vi "Custom PID v1_1.vi"(1 "Anti-Windup":bool, 2 "Set Point":dbl format="%.3g", 3 "Present Value":dbl format="%.3f", 4 "Tuning Parameters":T1={"Controller Gain, Kc"=1.0, "Reset Time, Ti (s)"=0.01, "Derivative Time, Td (s)"=0.0} {"Derivative Time, Td (s)" format="%.3g"; "Reset Time, Ti (s)" format="%.3g"; "Controller Gain, Kc" format="%.3g"}) -> (0 "Controller Output":dbl format="%.3g")   [LabVIEW 2012]
uses:
  Global Variables PID.vi
panel:
  out "dt (min)":dbl format="%.3g"
  in  "dT (s)":dbl=-1.0 step=0.001 format="%.3f"
  # "This PID VI is meant to be used for instructional Purposes.  It is in ideal form and simplified down from the orginal PID VI from the default NI PID VI."
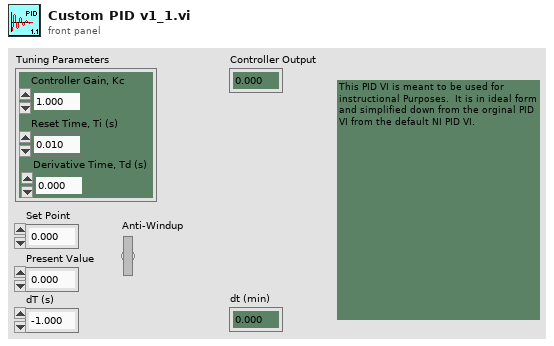
[diagram p1: front panel]
types:
  T1 = cluster{"Controller Gain, Kc":dbl, "Reset Time, Ti (s)":dbl, "Derivative Time, Td (s)":dbl}
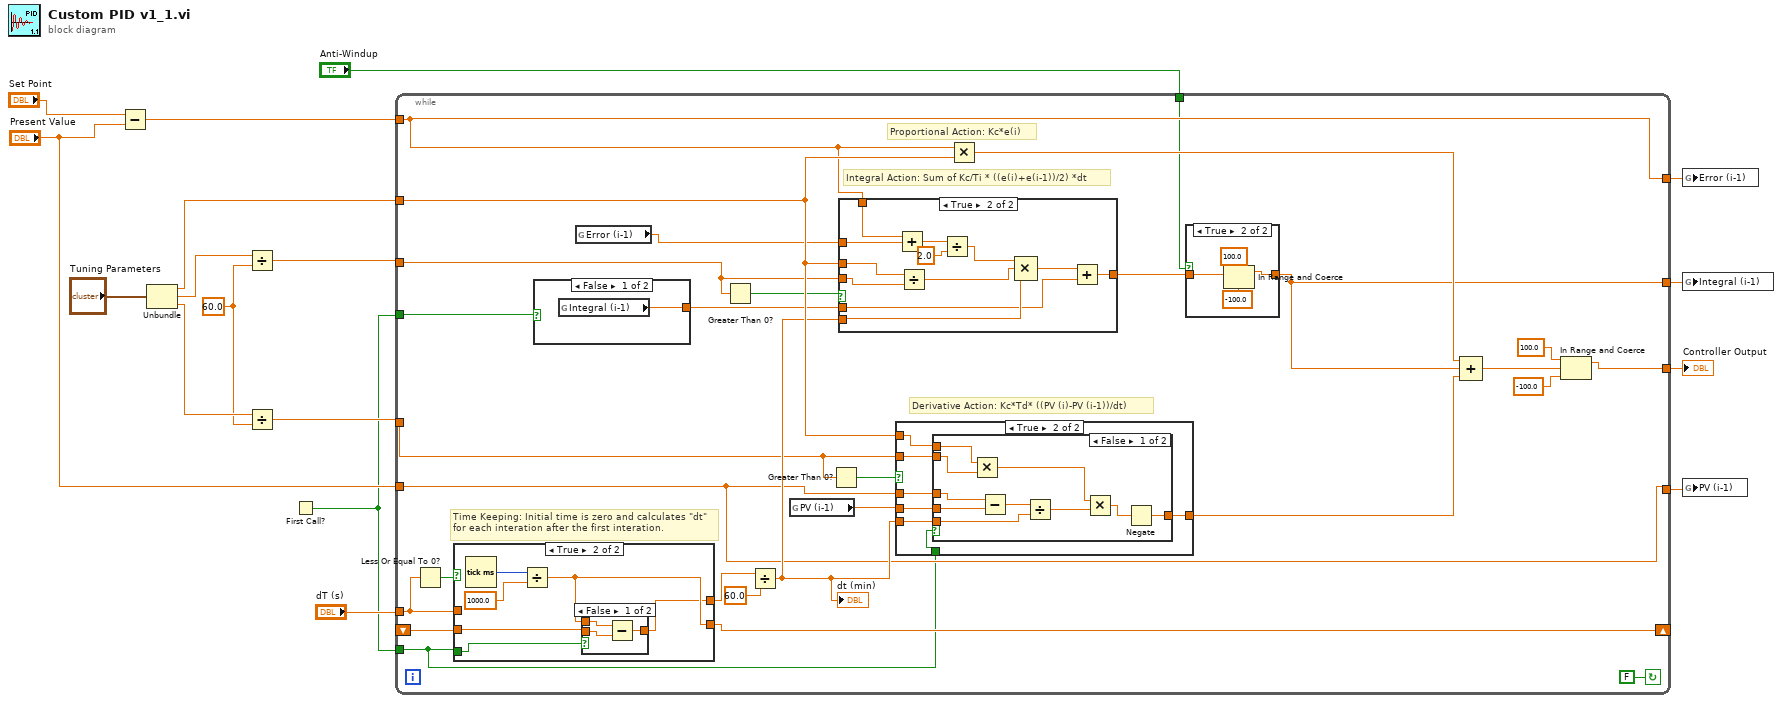
[diagram p0: block diagram]
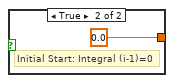
[diagram p3: hidden frame]
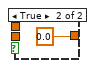
[diagram p5: hidden frame]
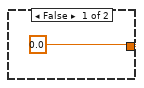
[diagram p6: hidden frame]
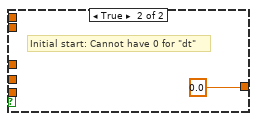
[diagram p7: hidden frame]
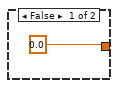
[diagram p8: hidden frame]
diagram:
  w8 = 60.0
  n1 = Subtract(x="Set Point", y="Present Value") -> (x-y=w16:dbl)
  n2 = Unbundle("Tuning Parameters") -> ("Controller Gain, Kc"=w12:dbl, "Reset Time, Ti (s)"=w14:dbl, "Derivative Time, Td (s)"=w13:dbl)
  n3 = Divide(x=w14, y=w8) -> (x/y=w11:dbl)
  n4 = Divide(x=w13, y=w8) -> (x/y=w10:dbl)
  n5 = First Call?() -> (First Call?: T/F=w5:bool)
  n6 = while {
    tunnel: w16 -> [w45]
    tunnel: w12 -> [w46]
    tunnel: w11 -> [w40]
    tunnel: w10 -> [w20]
    tunnel: w5 -> [w27]
    shift-right: [w36] -> _
    shift-left: _ -> [w44]
    tunnel: "dT (s)" -> [w42]
    tunnel: "Present Value" -> [w38]
    tunnel: [w30] -> w6
    tunnel: w5 -> [w26]
    tunnel: [w45] -> w4
    tunnel: [w19] -> w3
    tunnel: [w38] -> w2
    tunnel: "Anti-Windup" -> [w18]
    stop <- FALSE continue-if-true
    # "Derivative Action: Kc*Td* ((PV (i)-PV (i-1))/dt)"
    # "Proportional Action: Kc*e(i)"
    # "Integral Action: Sum of Kc/Ti * ((e(i)+e(i-1))/2) *dt"
    # "Time Keeping: Initial time is zero and calculates \"dt\" for each interation after the first interation."
    n7 = Less Or Equal To 0?(x=w42) -> (x <= 0?=w43:bool)
    n8 = case shown="True" w43 {
      tunnel: w27 -> [_ w60]
      tunnel: [w54 w57] -> w36
      tunnel: w44 -> [_ w58]
      tunnel: w42 -> [w54 _]
      tunnel: [w54 w55] -> w35
      frame False {
      }
      frame True {
        n9 = Tick Count (ms)() -> (millisecond timer value=w59:u32)
        n10 = Divide(x=w59, y=1000.0) -> (x/y=w57:dbl)
        n11 = case shown="False" w60 {
          tunnel: w57 -> [w63 _]
          tunnel: w58 -> [w62 _]
          tunnel: [w61 0.0] -> w55
          frame False {
            n12 = Subtract(x=w63, y=w62) -> (x-y=w61:dbl)
          }
          frame True {
          }
        }
      }
    }
    n13 = case shown="False" w26 {
      tunnel: [w52 0.0] -> w25
      frame False {
        n14 = global read "Global Variables PID.vi" "Integral (i-1)"() -> (w52:dbl)
      }
      frame True {
        # "Initial Start: Integral (i-1)=0"
      }
    }
    n15 = global read "Global Variables PID.vi" "Error (i-1)"() -> (w22:dbl)
    n16 = Greater Than 0?(x=w40) -> (x > 0?=w39:bool)
    n17 = Divide(x=w35, y=60.0) -> (x/y=w41:dbl)
    "dt (min)" <- w41
    n18 = global read "Global Variables PID.vi" "PV (i-1)"() -> (w21:dbl)
    n19 = Greater Than 0?(x=w20) -> (x > 0?=w29:bool)
    n20 = case shown="True" w39 {
      tunnel: w46 -> [_ w92]
      tunnel: w40 -> [_ w91]
      tunnel: w22 -> [_ w93]
      tunnel: w45 -> [_ w94]
      tunnel: w41 -> [_ w88]
      tunnel: [0.0 w86] -> w23
      tunnel: w25 -> [_ w85]
      frame False {
      }
      frame True {
        n21 = Add(x=w94, y=w93) -> (x+y=w96:dbl)
        n22 = Divide(x=w92, y=w91) -> (x/y=w89:dbl)
        n23 = Divide(x=w96, y=2.0) -> (x/y=w90:dbl)
        n24 = Compound Arithmetic op=MULTIPLY(w90, w89, w88) -> (w87:dbl)
        n25 = Add(x=w87, y=w85) -> (x+y=w86:dbl)
      }
    }
    n26 = case shown="True" w29 {
      tunnel: w46 -> [_ w69]
      tunnel: w20 -> [_ w68]
      tunnel: w41 -> [_ w70]
      tunnel: w38 -> [_ w72]
      tunnel: w21 -> [_ w71]
      tunnel: [0.0 w67] -> w37
      tunnel: w27 -> [_ w66]
      frame False {
      }
      frame True {
        n27 = case shown="False" w66 {
          tunnel: w72 -> [w82 _]
          tunnel: w71 -> [w81 _]
          tunnel: w70 -> [w79 _]
          tunnel: w69 -> [w78 _]
          tunnel: w68 -> [w77 _]
          tunnel: [w73 0.0] -> w67
          frame False {
            n28 = Multiply(x=w78, y=w77) -> (x*y=w76:dbl)
            n29 = Subtract(x=w82, y=w81) -> (x-y=w80:dbl)
            n30 = Divide(x=w80, y=w79) -> (x/y=w75:dbl)
            n31 = Multiply(x=w76, y=w75) -> (x*y=w74:dbl)
            n32 = Negate(x=w74) -> (-x=w73:dbl)
          }
          frame True {
            # "Initial start: Cannot have 0 for \"dt\""
          }
        }
      }
    }
    n33 = Multiply(x=w45, y=w46) -> (x*y=w24:dbl)
    n34 = case shown="True" w18 {
      tunnel: w23 -> [w47 w51]
      tunnel: [w47 w50] -> w19
      frame False {
      }
      frame True {
        n35 = In Range and Coerce(upper limit=100.0 ("lower limit"), x=w51, lower limit=-100.0) -> (coerced(x)=w50:dbl)  [unwired: 1 out]
      }
    }
    n36 = Compound Arithmetic op=ADD(w24, w19, w37) -> (w31:dbl)
    n37 = In Range and Coerce(upper limit=100.0 ("x"), x=w31, lower limit=-100.0 ("x")) -> (coerced(x)=w30:dbl)  [unwired: 1 out]
  }
  "Controller Output" <- w6
  n38 = global write "Global Variables PID.vi" "Error (i-1)"(w4) -> ()
  n39 = global write "Global Variables PID.vi" "Integral (i-1)"(w3) -> ()
  n40 = global write "Global Variables PID.vi" "PV (i-1)"(w2) -> ()
